vi "Start Trial.vi"(8 "error in (no error)":errorcluster, 10 "Trial Number":i32, 11 "Accelerometer in":refnum<class "Accelerometer.lvclass">) -> (0 "error out":errorcluster, 3 "Accelerometer out":refnum<class "Accelerometer.lvclass">)   [LabVIEW 2020, in "Accelerometer.lvlib" / "Accelerometer.lvclass"]
uses:
  Accelerometer.lvclass
  Accelerometer.lvclass/Accelerometer.ctl
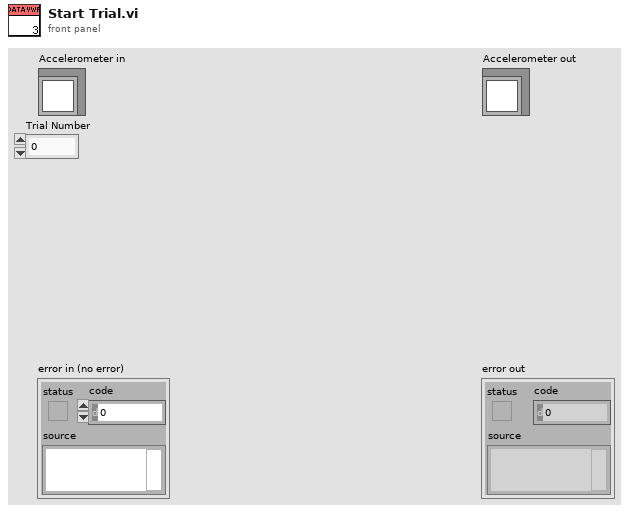
[diagram p1: front panel]
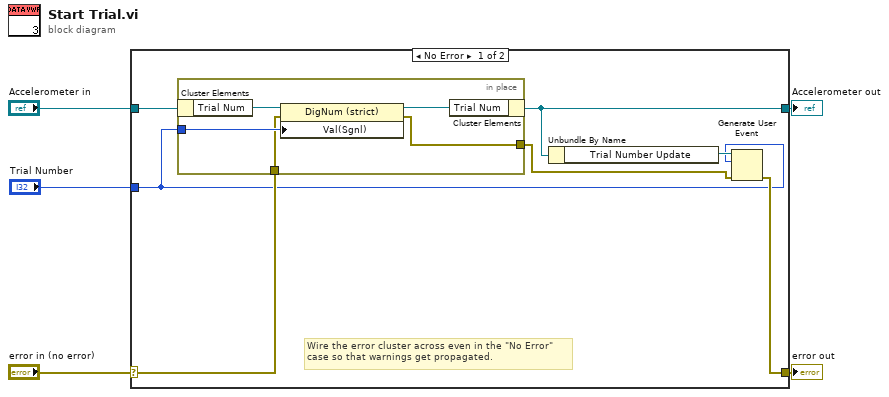
[diagram p0: block diagram]
diagram:
  n1 = case shown="No Error" "error in (no error)" {
    selector: "error in (no error)" -> [w7 w19]
    tunnel: [w8 w19] -> w4
    tunnel: [w9 w18] -> w2
    tunnel: "Accelerometer in" -> [w10 w18]
    tunnel: "Trial Number" -> [w6 _]
    frame No Error {
      # "Wire the error cluster across even in the \"No Error\"\ncase so that warnings get propagated."
      n2 = in-place {
        in-place-border: w6 -> [w15]
        in-place-border: [w14] -> w11
        in-place-border: w7 -> [w13]
        n3 = in-place-cluster #1(w10) -> ("Trial Num"=w17:refnum<vi>)
        n4 = property class="DigNum (strict)"(reference=w17, error in=w13, "Val(Sgnl)"=w15) -> (reference out=w16:refnum<vi>, error out=w14:errorcluster)
        n5 = in-place-cluster #1("Trial Num"=w16) -> (w9:refnum<class "Accelerometer.lvclass">)
      }
      n6 = Unbundle By Name(w9) -> ("Trial Number Update"=w12:refnum<user-event>)
      n7 = Generate User Event(user event=w12, event data cluster=w6, error in=w11) -> (error out=w8:errorcluster)  [unwired: 1 in, 1 out]
    }
    frame Error {
    }
  }
  "error out" <- w4
  "Accelerometer out" <- w2
